vi "_Test Method Hanging.vi"(8 "error in (no error)":errorcluster, 11 "Hanging Demo Case 2 In":refnum<class "Hanging Dummy Case 2.lvclass">) -> (0 "error out":errorcluster, 3 "Hanging Demo Case 2 Out":refnum<class "Hanging Dummy Case 2.lvclass">)   [LabVIEW 2020, in "Hanging Dummy Case 2.lvclass"]
uses:
  Hanging Dummy Case 2.lvclass
  C:/Git/astemes-lunit/source/Framework/Test Case/LUnit Test Case.lvclass
  source/Framework/Test Case/LUnit Test Case.lvclass/LUnit Test Case.ctl
  source/Framework/Test Case/Private/SubVIs/Add test result.vi
  source/Framework/Test Case/Private/SubVIs/Set Assertion Type.vi
  source/Framework/Result Types/Case Result/Public/Record Assertion Result.vi
  source/Framework/Result Types/Method Result/Public/Aggregate Assertion Results.vi
  source/Framework/Result Types/Method Result/Private/Merge Status.vi
  source/Framework/Result Types/Method Result/Private/Concatenate result strings.vi
  source/Framework/Test Case/LUnit Test Case.lvclass
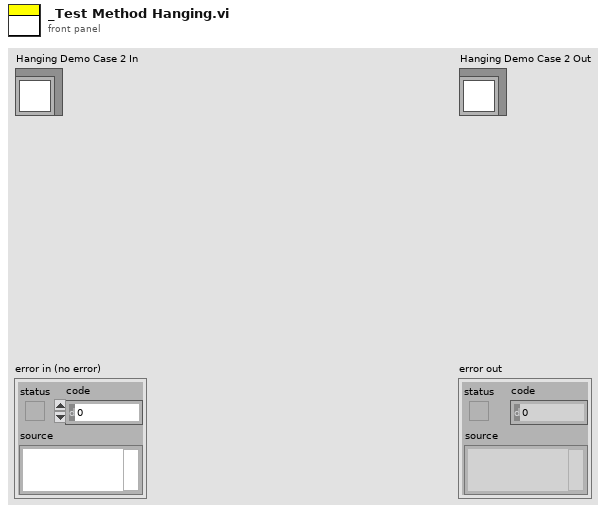
[diagram p1: front panel]
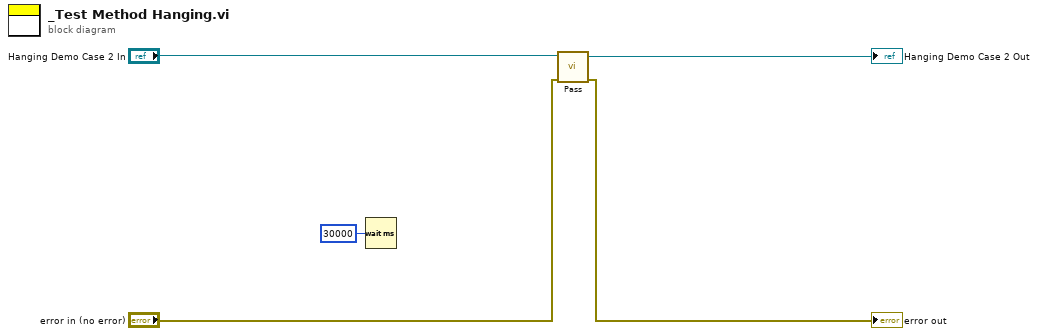
[diagram p0: block diagram]
diagram:
  n1 = Wait (ms)(milliseconds to wait=u32 30000) -> ()  [unwired: 1 out]
  n2 = call "Pass.vi"("error in (no error)"="error in (no error)", "LUnit Test Case In"="Hanging Demo Case 2 In") -> ("error out"=→"error out":errorcluster, "LUnit Test Case Out"=→"Hanging Demo Case 2 Out":refnum<class "Hanging Dummy Case 2.lvclass">)  [unwired: 8 in]
